vi "testing_simple_motor_on.vi"() -> ()   [LabVIEW 2019]
uses:
  simple_on.ctl
  <vilib>/Rock Robotics/WPI/RobotDrive/WPI_RobotDriveArcadeDrive_Standard(NoSaturation).vi
  <vilib>/Rock Robotics/Network Tables/NT Write Numeric Array.vi
panel:
  in  "Motor On Time":dbl
  out "Motor State":T1
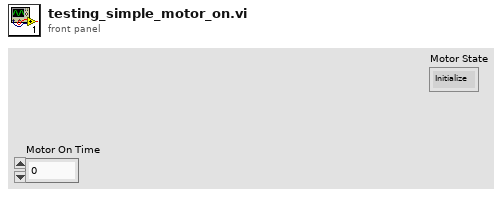
[diagram p1: front panel]
types:
  T1 = typedef "simple_on.ctl" = enum16{"Initialize", "Start Motor", "Countdown", "Stop Motor"}
  T2 = typedef "WPI_RobotDriveDevRef.ctl" = cluster{"DevStatus":errorcluster, "Motors[]":T3[], "Square Inputs":bool, "Max Output":dbl}
  T3 = typedef "WPI_MotorControlDeviceRef.ctl" = cluster{"DeviceStatus":errorcluster, "Type":T4, "PWM":cluster{"PWM Channel":T5, "DeadBand":T6}, "CAN":cluster{"Device Number":u8, "SetOutput VI Ref":variant, "GetOutput VI Ref":variant, "Enable VI Ref":variant, "Disable VI Ref":variant, "Data":variant}, "Invert":bool, "DIO PWM":cluster{"PWM \"Enable\" Channel":T5, "DIOChannel":T7, "PWM Rate":dbl}}
  T4 = typedef "WPI_MotorControlType.ctl" = enum16{"PWM", "CAN", "DIO PWM"}
  T5 = typedef "FPGA_DIOPWMChannel.ctl" = enum8{"PWM 0", "PWM 1", "PWM 2", "PWM 3", "PWM 4", "PWM 5", "PWM 6", "PWM 7", "PWM 8", "PWM 9", "PWM MXP 0", "PWM MXP 1", "PWM MXP 2", "PWM MXP 3", "PWM MXP 4", "PWM MXP 5", "PWM MXP 6", "PWM MXP 7", "PWM MXP 8", "PWM MXP 9", "Invalid"}
  T6 = typedef "WPI_PWMDeadband.ctl" = cluster{"Name":string, "maxPositivePwm":i32, "minPositivePwm":i32, "centerPwm":i32, "maxNegativePwm":i32, "minNegativePwm":i32, "angularRange":u16}
  T7 = typedef "FPGA_DIOChannel.ctl" = enum8{"DIO 0", "DIO 1", "DIO 2", "DIO 3", "DIO 4", "DIO 5", "DIO 6", "DIO 7", "DIO 8", "DIO 9", "DIO MXP 0", "DIO MXP 1", "DIO MXP 2", "DIO MXP 3", "DIO MXP 4", "DIO MXP 5", "DIO MXP 6", "DIO MXP 7", "DIO MXP 8", "DIO MXP 9", "DIO MXP 10", "DIO MXP 11", "DIO MXP 12", "DIO MXP 13", "DIO MXP 14", "DIO MXP 15", "SPI Port CS1", "SPI Port CS2", "SPI Port CS3", "SPI Port MISO", "SPI Port MOSI", "Invalid"}
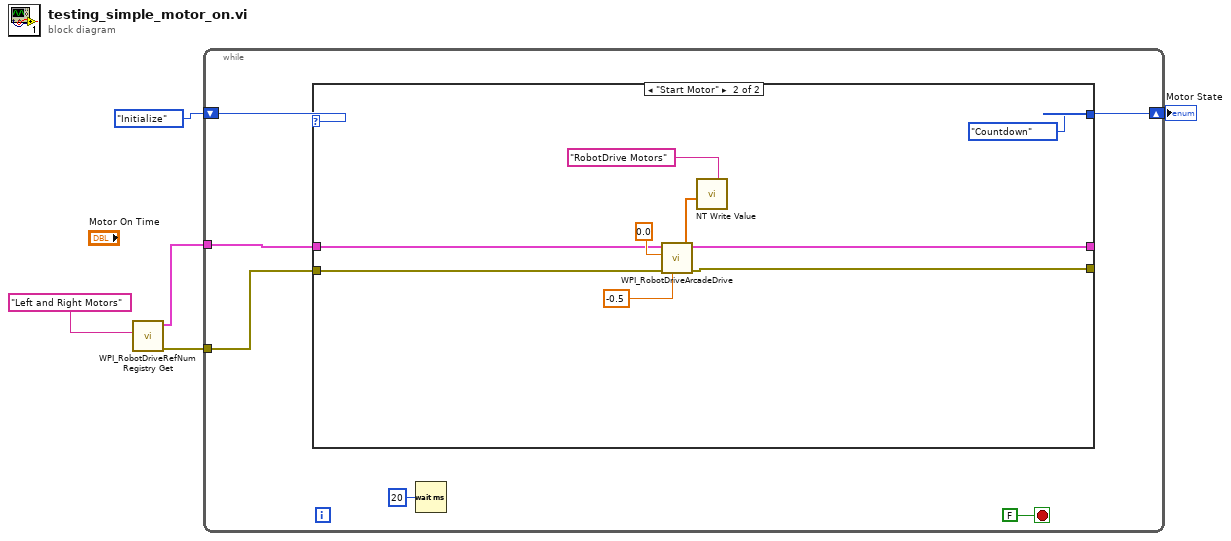
[diagram p0: block diagram]
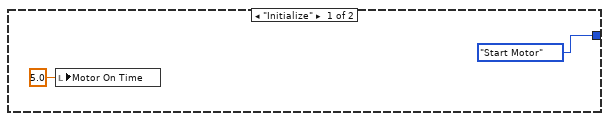
[diagram p2: hidden frame]
diagram:
  n1 = call <vilib>:"WPI_RobotDriveRefNum Registry Get.vi"("refnum name"="Left and Right Motors") -> ("error out"=w1:errorcluster, "RobotDriveDevRef"=w2:T2)  [unwired: 9 in]
  n2 = while {
    shift-right: [w8] -> w4
    shift-left: simple_on."Initialize" ("Enum") -> [w9]
    tunnel: w2 -> [w7]
    tunnel: w1 -> [w6]
    stop <- FALSE stop-if-true
    n3 = case shown="\"Start Motor\"" w9 {
      tunnel: [simple_on."Start Motor" ("Enum") simple_on."Countdown" ("Enum")] -> w8
      tunnel: w7 -> [_ w17]
      tunnel: w6 -> [_ w16]
      tunnel: [_ w15] -> _
      tunnel: [_ w14] -> _
      frame "Initialize" {
        n4 = local write "Motor On Time"(5.0 ("Motor On Time")) -> ()
      }
      frame "Start Motor" {
        n5 = call-poly <vilib>:"WPI_RobotDriveArcadeDrive.vi"("error in (no error)"=w16, "Y axis value"=-0.5, "X axis value"=0.0, "RobotDriveDevRef"=w17) -> ("error out"=w14:errorcluster, "Motor Values"=w21:dbl[], "RobotDriveDevRef"=w15:T2)  [unwired: 5 out]
        n6 = call-poly <vilib>:"NT Write Value.vi"("Numeric Array"=w21, "Name"="RobotDrive Motors") -> ()  [unwired: 9 in, 1 out]
      }
    }
    n7 = Wait (ms)(milliseconds to wait=u32 20) -> ()  [unwired: 1 out]
  }
  "Motor State" <- w4
